vi "TransformString.vi"(8 "error in (no error)":errorcluster, 10 "String":string, 11 "LogicalNot in":refnum<class "LogicalNot.lvclass">) -> (0 "error out":errorcluster, 2 "String out":string, 3 "LogicalNot out":refnum<class "LogicalNot.lvclass">)   [LabVIEW 2019, in "Constraint.lvlib" / "LogicalNot.lvclass"]
doc: "Transforms the string returned by the member constraint's <B>ToString</B> or <B>FailureDescription</B> such that it reflects the operation of this expression."
uses:
  LogicalNot.lvclass
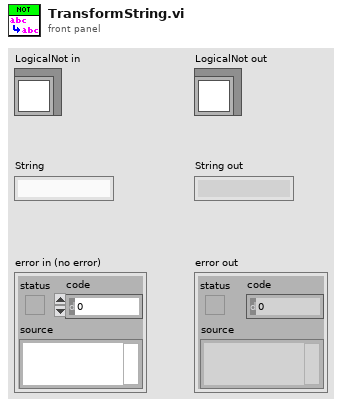
[diagram p1: front panel]
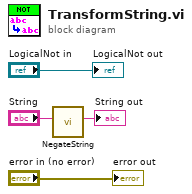
[diagram p0: block diagram]
diagram:
  n1 = call "NegateString.vi"("String"="String") -> ("Negated String"=→"String out":string)  [unwired: 10 in]
  "error out" <- "error in (no error)"
  "LogicalNot out" <- "LogicalNot in"
